vi "Motor Saftey.vi"() -> (0 "Motor Saftey":T1)   [LabVIEW 2014]
uses:
  <vilib>/Rock Robotics/WPI/SafetyOutput/WPI_SafetyOutputConfigMenu.ctl
  <vilib>/Rock Robotics/Network Tables/SD Read Boolean.vi
  <vilib>/Rock Robotics/Network Tables/SD Write Boolean.vi
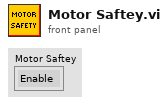
[diagram p1: front panel]
types:
  T1 = typedef "WPI_SafetyOutputConfigMenu.ctl" = enum16{"Enable", "Disable"}
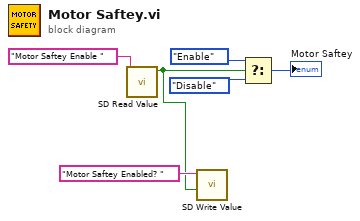
[diagram p0: block diagram]
diagram:
  n1 = call-poly <vilib>:"SD Read Value.vi"("Name"="Motor Saftey Enable ") -> ("Boolean"=w1:bool)  [unwired: 8 in, 2 out]
  n2 = call-poly <vilib>:"SD Write Value.vi"("Boolean"=w1, "Name"="Motor Saftey Enabled? ") -> ()  [unwired: 8 in, 2 out]
  n3 = Select(t=WPI_SafetyOutputConfigMenu."Enable" ("mode"), s=w1, f=WPI_SafetyOutputConfigMenu."Disable" ("mode")) -> (s? t:f=→"Motor Saftey":T1)
